vi "Read any file TDMS 1chan only.vi"(7 "tdms file in":refnum<k34>, 8 "error in":errorcluster, 9 "Data File Type":T2(ring), 10 "Data window":T1={"Start"=0, "Length"=500000, "Channel numbers"=[0], "Channel name"="", "Group name"="Untitled"}, 11 "Input file path":path) -> (0 "error out":errorcluster, 1 "1st channel length":u64, 2 "Data out":waveform(dbl), 3 "Actual input file path":path, 5 "tdms file out":refnum<k34>)   [LabVIEW 2015]
panel:
  # "OR"
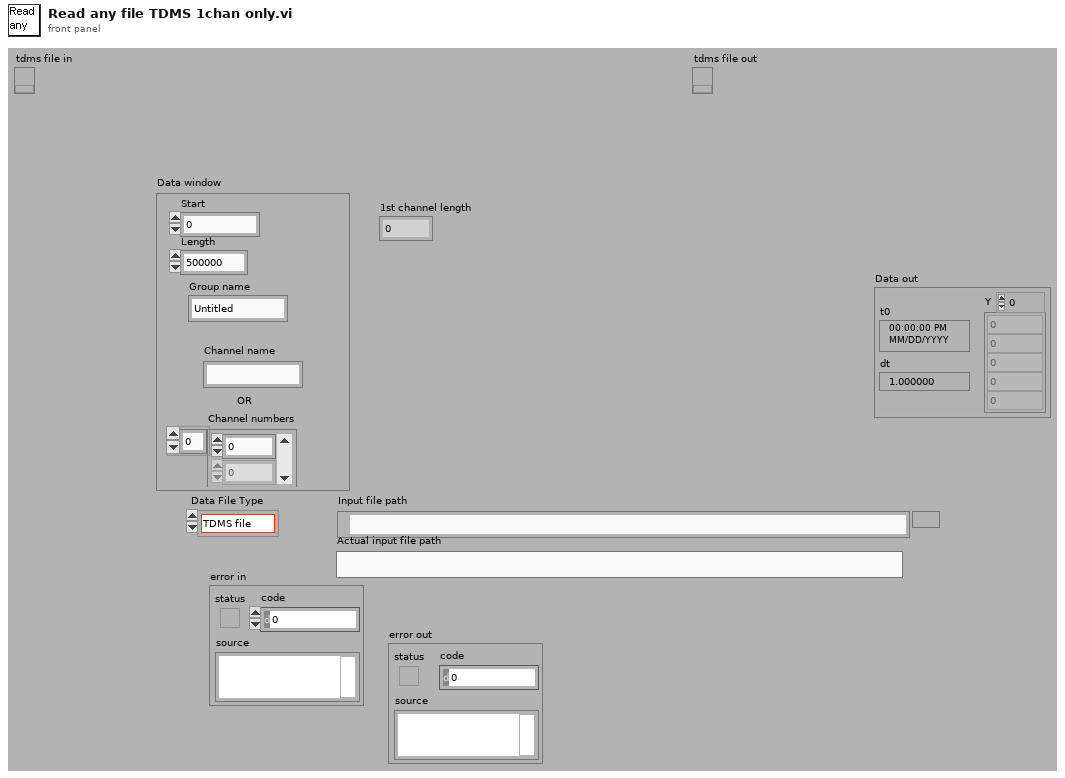
[diagram p1: front panel]
types:
  T1 = cluster{"Start":i64, "Length":i32, "Channel numbers":i64[], "Channel name":string, "Group name":string}
  T2 = enum16{"TDMS file", "Tektronics ISF", "BinF file", "ASCII File", "BinH File", "BinW File", "BINARY File"}
  T3 = enum16{"open", "open or create", "create or replace", "create", "open (read-only)"}
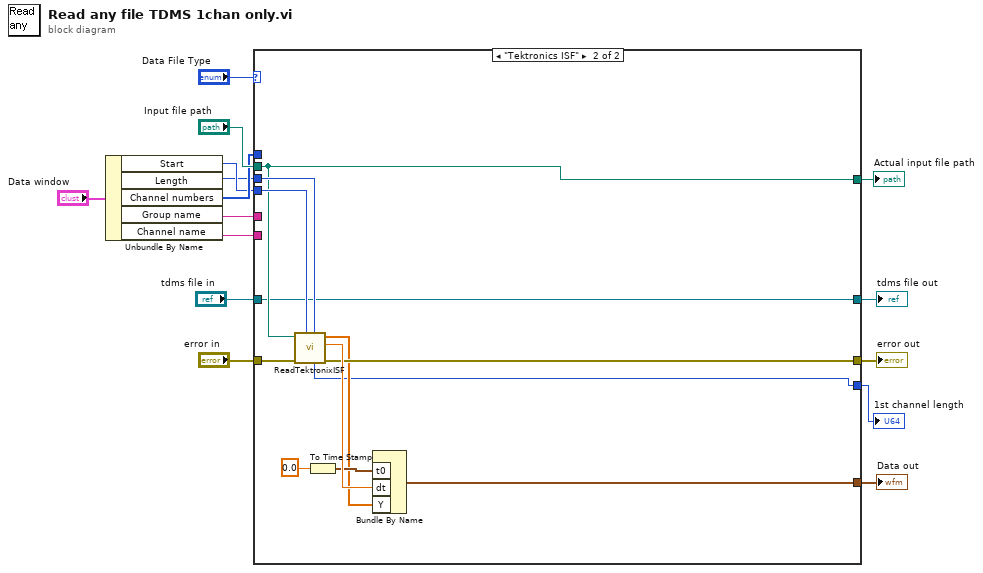
[diagram p0: block diagram]
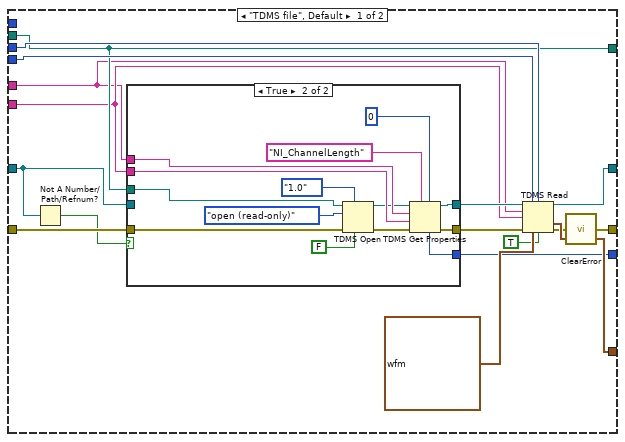
[diagram p2: hidden frame]
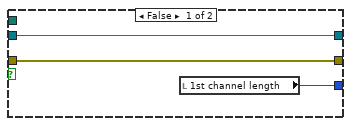
[diagram p3: hidden frame]
diagram:
  n1 = Unbundle By Name("Data window") -> ("Start"=w10:i64, "Length"=w9:i32, "Channel numbers"=w11:i64[], "Group name"=w6:string, "Channel name"=w8:string)
  n2 = case shown="\"Tektronics ISF\"" "Data File Type" {
    tunnel: "Input file path" -> [w27 w53]
    tunnel: [w27 w53] -> w13
    tunnel: "error in" -> [w32 w56]
    tunnel: [w21 w55] -> w4
    tunnel: w11 -> [_ _]
    tunnel: w10 -> [w29 w57]
    tunnel: w9 -> [w28 w58]
    tunnel: [w22 w51] -> w1
    tunnel: w8 -> [w19 _]
    tunnel: [w20 w52] -> w7
    tunnel: w6 -> [w18 _]
    tunnel: [w25 w50] -> w3
    tunnel: "tdms file in" -> [w23 w50]
    frame "TDMS file", Default {
      n3 = Not A Number/Path/Refnum?(number/path/refnum=w23) -> (NaN/Path/Refnum?=w24:bool)
      n4 = case shown="True" w24 {
        tunnel: w32 -> [w34 w49]
        tunnel: [w35 w38] -> w31
        tunnel: [w34 w43] -> w30
        tunnel: w27 -> [_ w48]
        tunnel: w23 -> [w35 _]
        tunnel: [w33 w42] -> w20
        tunnel: w19 -> [_ w41]
        tunnel: w18 -> [_ w40]
        frame False {
          n5 = local read "1st channel length"() -> (w33:u64)
        }
        frame True {
          n6 = TDMS Open(6:FALSE ("disable buffering (T)"), 7:enum16{"1.0", "2.0"}."1.0" ("file format version (2.0)"), 8:w49, 10:T3."open (read-only)" ("operation (0:open)"), 11:w48) -> (0:w44:errorcluster, 3:w39:refnum<k34>)  [unwired: 2 in]
          n7 = TDMS Get Properties(5:u64 0, 7:"NI_ChannelLength" ("property name"), 8:w44, 9:w41, 10:w40, 11:w39) -> (0:w43:errorcluster, 3:w38:refnum<k34>, 4:w42:u64)  [unwired: 3 out]
        }
      }
      n8 = TDMS Read(0:w31, 1:w29, 2:w28, 5:w18, 7:w19, 11:w30, 12:waveform(dbl) {"t0"=timestamp(0 s since 1904-01-01), "dt"=1.0, "Y"=[]}, 13:TRUE ("return channels in file order? (F)")) -> (4:w25:refnum<k34>, 10:w22:waveform(dbl), 15:w17:errorcluster)  [unwired: 3 out]
      n9 = call <vilib>:"ClearError.vi"("error in (no error)"=w17) -> ("error out"=w21:errorcluster)
    }
    frame "Tektronics ISF" {
      n10 = call "ReadTektronixISF.vi"("Length"=w58, "Start"=w57, "error in (no error)"=w56, "Path"=w53) -> ("error out"=w55:errorcluster, "dt"=w61:dbl, "Data"=w54:dbl[], "Total number of points"=w52:u64)  [unwired: 4 out]
      n11 = To Time Stamp(1:0.0) -> (0:w59:timestamp)
      n12 = Bundle By Name("t0"=w59, "dt"=w61, "Y"=w54) -> (w51:waveform(dbl))  [unwired: 1 out]
    }
  }
  "Actual input file path" <- w13
  "error out" <- w4
  "1st channel length" <- w7
  "tdms file out" <- w3
  "Data out" <- w1
